vi "Check Device IDs are Temperature Devices.vi"(8 "error in":errorcluster, 11 "Mercury Reference In":T1) -> (0 "error out":errorcluster, 2 "Valid?":bool, 3 "Mercury Reference Out":T1)   [LabVIEW 2013, in "Mercury iXX.lvlib" / "Control Loop.lvlib"]
uses:
  <instrlib>/Mercury iXX/Public/Libraries/Control Loop.lvlib
  <instrlib>/Mercury iXX/Public/Controls/Mercury Reference.ctl
  <instrlib>/Mercury iXX/Public/Controls/Comms Transport Layer.ctl
  <instrlib>/Mercury iXX/Private/Controls/Query Dynamic Reference.ctl
  <vilib>/regexp/Match Regular Expression.xnode
  <instrlib>/Mercury iXX/Mercury iXX.lvlib
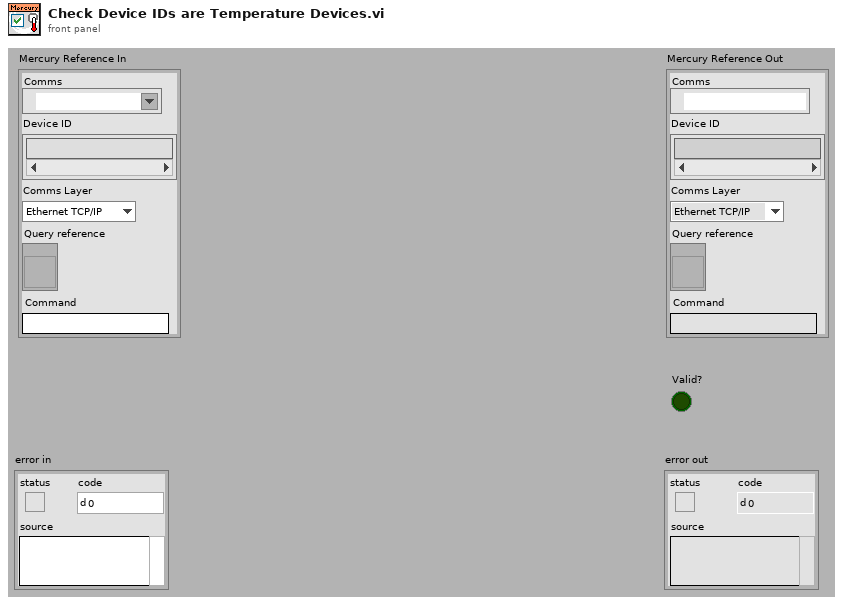
[diagram p1: front panel]
types:
  T1 = typedef "Mercury iXX.lvlib/Mercury Reference.ctl" = cluster{"Comms":refnum<visa-resource-name>, "Device ID":string[], "Comms Layer":T2, "Command":string, "Query reference":T3}
  T2 = typedef "Mercury iXX.lvlib/Comms Transport Layer.ctl" = enum16{"Ethernet TCP/IP", "USB", "ISOBus - RS-232", "GPIB"}
  T3 = typedef "Mercury iXX.lvlib/Query Dynamic Reference.ctl" = refnum<vi>
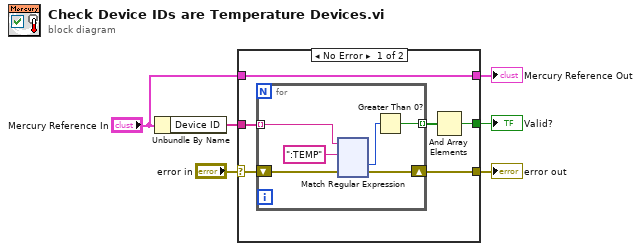
[diagram p0: block diagram]
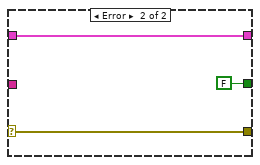
[diagram p2: hidden frame]
diagram:
  n1 = Unbundle By Name("Mercury Reference In") -> ("Device ID"=w3:string[])
  n2 = case shown="No Error" "error in" {
    selector: "error in" -> [w10 w135]
    tunnel: [w9 w135] -> w5
    tunnel: w3 -> [w8 _]
    tunnel: [w11 FALSE] -> w4
    tunnel: "Mercury Reference In" -> [w7 w133]
    tunnel: [w7 w133] -> w1
    frame No Error {
      n3 = for {
        tunnel: w8 -> [w18] mode=indexing
        tunnel: [w15] -> w12 mode=indexing
        shift-right: [w13] -> w9
        shift-left: w10 -> [w14]
        n4 = xnode "Match Regular Expression"("input string"=w18, "regular expression"=":TEMP", "error in"=w14) -> ("offset past match"=w16:i32, "error out"=w13:errorcluster)  [unwired: 1 in, 5 out]
        n5 = Greater Than 0?(x=w16) -> (x > 0?=w15:bool)
      }
      n6 = And Array Elements(Boolean array=w12) -> (logical AND=w11:bool)
    }
    frame Error {
    }
  }
  "error out" <- w5
  "Valid?" <- w4
  "Mercury Reference Out" <- w1
